vi "Vision 차선, 표지판 통합.vi"() -> ()   [LabVIEW 2016]
uses:
  <vilib>/vision/NI_Vision_Development_Module.lvlib
  <vilib>/ptbypt/NI_PtbyPt.lvlib
  <vilib>/vision/Classification.llb/IMAQ Classifier Nearest Neighbor options.ctl
panel:
  out "출력 클러스터":T1
  out "ms 타이머 값":u32
  in  "정적 횟수":u8
  in  "동적 횟수":u8
  in  "유턴 횟수":u8
  in  "Stop (F) 2":bool caption="Stop (F)"
  out "유턴이냐":bool
  in  "Type":u32(ring)=3 items=["No Selection", "Point", "Line", "Rectangle", "Oval", "Polygon", "Free", "Annulus", "Unused2", "Unused3", "Broken Line", "Free Hand Line", "Rotated Rectangle"]
  in  "ID":enum32{"External", "Internal"}(ring)
  out "동적이냐":bool
  out "정적이냐":bool
  in  "탭 컨트롤":enum32{"유턴", "동적", "정적"}(tab)
  in  "Paramaters":T3={"Preprocessing Options"={"Method"=-1, "Looking for"=1, "Threshold Range"={"Lower value"=0.0, "Upper value"=69.0}, "Threshold Limits"={"Lower value"=0.0, "Upper value"=0.0}, "Reject Border"=FALSE, "# of Erosions"=0, "Kernel Size"={"Lower value"=0, "Upper value"=0}, "Deviation Factor"=0.0}, "Nearest Neighbor Options"={"Method"=0, "Metric"=0, "k"=0}, "Particle Options"={"Scale Dependant"=FALSE, "Scale Factor"=0.0, "Symmetry Dependant"=FALSE, "Symmetry Factor"=0.0}} {"Preprocessing Options"."Deviation Factor" min=0.0; "Preprocessing Options"."Threshold Limits"."Upper value" format="%.2f"; "Preprocessing Options"."Threshold Limits"."Lower value" format="%.2f"; "Preprocessing Options"."Threshold Range"."Upper value" format="%.2f"; "Preprocessing Options"."Threshold Range"."Lower value" format="%.2f"; "Preprocessing Options"."# of Erosions" min=0; "Preprocessing Options"."Method" items=["Manual Threshold"=-1, "-"=-2, "Auto Threshold: Clustering"=0, "Auto Threshold: Entropy"=1, "Auto Threshold: Metric"=2, "Auto Threshold: Moments"=3, "Auto Threshold: Inter-class Variance"=4, "--"=-3, "Local Threshold: Niblack"=5, "Local Threshold: BG Correction"=6]; "Preprocessing Options"."Looking for" items=["Bright Objects", "Dark Objects"]; "Nearest Neighbor Options"."Method" items=["Nearest Neighbor", "K Nearest Neighbor", "Minimum Mean Distance"]; "Nearest Neighbor Options"."Metric" items=["Maximum", "Sum", "Euclidean"]; "Nearest Neighbor Options"."k" min=3}
  in  "Paramaters 2":T3={"Preprocessing Options"={"Method"=-1, "Looking for"=0, "Threshold Range"={"Lower value"=0.0, "Upper value"=45.0}, "Threshold Limits"={"Lower value"=0.0, "Upper value"=0.0}, "Reject Border"=FALSE, "# of Erosions"=0, "Kernel Size"={"Lower value"=0, "Upper value"=0}, "Deviation Factor"=0.0}, "Nearest Neighbor Options"={"Method"=0, "Metric"=0, "k"=0}, "Particle Options"={"Scale Dependant"=FALSE, "Scale Factor"=0.0, "Symmetry Dependant"=FALSE, "Symmetry Factor"=0.0}} {"Preprocessing Options"."Deviation Factor" min=0.0; "Preprocessing Options"."Threshold Limits"."Upper value" format="%.2f"; "Preprocessing Options"."Threshold Limits"."Lower value" format="%.2f"; "Preprocessing Options"."Threshold Range"."Upper value" format="%.2f"; "Preprocessing Options"."Threshold Range"."Lower value" format="%.2f"; "Preprocessing Options"."# of Erosions" min=0; "Preprocessing Options"."Method" items=["Manual Threshold"=-1, "-"=-2, "Auto Threshold: Clustering"=0, "Auto Threshold: Entropy"=1, "Auto Threshold: Metric"=2, "Auto Threshold: Moments"=3, "Auto Threshold: Inter-class Variance"=4, "--"=-3, "Local Threshold: Niblack"=5, "Local Threshold: BG Correction"=6]; "Preprocessing Options"."Looking for" items=["Bright Objects", "Dark Objects"]; "Nearest Neighbor Options"."Method" items=["Nearest Neighbor", "K Nearest Neighbor", "Minimum Mean Distance"]; "Nearest Neighbor Options"."Metric" items=["Maximum", "Sum", "Euclidean"]; "Nearest Neighbor Options"."k" min=3}
  in  "Paramaters 3":T3={"Preprocessing Options"={"Method"=-1, "Looking for"=0, "Threshold Range"={"Lower value"=0.0, "Upper value"=45.0}, "Threshold Limits"={"Lower value"=0.0, "Upper value"=0.0}, "Reject Border"=FALSE, "# of Erosions"=0, "Kernel Size"={"Lower value"=0, "Upper value"=0}, "Deviation Factor"=0.0}, "Nearest Neighbor Options"={"Method"=0, "Metric"=0, "k"=0}, "Particle Options"={"Scale Dependant"=FALSE, "Scale Factor"=0.0, "Symmetry Dependant"=FALSE, "Symmetry Factor"=0.0}} {"Preprocessing Options"."Deviation Factor" min=0.0; "Preprocessing Options"."Threshold Limits"."Upper value" format="%.2f"; "Preprocessing Options"."Threshold Limits"."Lower value" format="%.2f"; "Preprocessing Options"."Threshold Range"."Upper value" format="%.2f"; "Preprocessing Options"."Threshold Range"."Lower value" format="%.2f"; "Preprocessing Options"."# of Erosions" min=0; "Preprocessing Options"."Method" items=["Manual Threshold"=-1, "-"=-2, "Auto Threshold: Clustering"=0, "Auto Threshold: Entropy"=1, "Auto Threshold: Metric"=2, "Auto Threshold: Moments"=3, "Auto Threshold: Inter-class Variance"=4, "--"=-3, "Local Threshold: Niblack"=5, "Local Threshold: BG Correction"=6]; "Preprocessing Options"."Looking for" items=["Bright Objects", "Dark Objects"]; "Nearest Neighbor Options"."Method" items=["Nearest Neighbor", "K Nearest Neighbor", "Minimum Mean Distance"]; "Nearest Neighbor Options"."Metric" items=["Maximum", "Sum", "Euclidean"]; "Nearest Neighbor Options"."k" min=3}
  in  "탭 컨트롤 2":enum32{"유턴", "동적", "정적"}(tab)
  in  "File Path":path=path "C:/Users/SeongHyeon/Desktop/전체프로그램/Sub Vi/Sensor/Vision Reference/유턴.clf"
  in  "File Path 2":path=path "C:/Users/SeongHyeon/Desktop/전체프로그램/Sub Vi/Sensor/Vision Reference/동적.clf"
  in  "File Path 3":path=path "C:/Users/SeongHyeon/Desktop/전체프로그램/Sub Vi/Sensor/Vision Reference/정적.clf"
  in  "탭 컨트롤 3":enum32{"유턴", "동적", "정적"}(tab)
  out "유턴":T4(plugin-control)
  out "동적":T4(plugin-control)
  out "정적":T4(plugin-control)
  out "횡단보도 거리":dbl[](array[numeric])
  out "차선":dbl[][](array[numeric])
  out "Filtered image":T4(plugin-control)
  out "Original Image":T4(plugin-control)
  out "Original Image":T4(plugin-control)
  out "프레임 rate":dbl
  out "error out":errorcluster
  in  "이미지 형식":T5 items=["Grayscale (U8)", "Grayscale (I16)", "Grayscale (SGL)", "Complex (CSG)", "RGB (U32)", "HSL (U32)", "RGB (U64)", "Grayscale (U16)"]
  in  "Stop (F)":bool
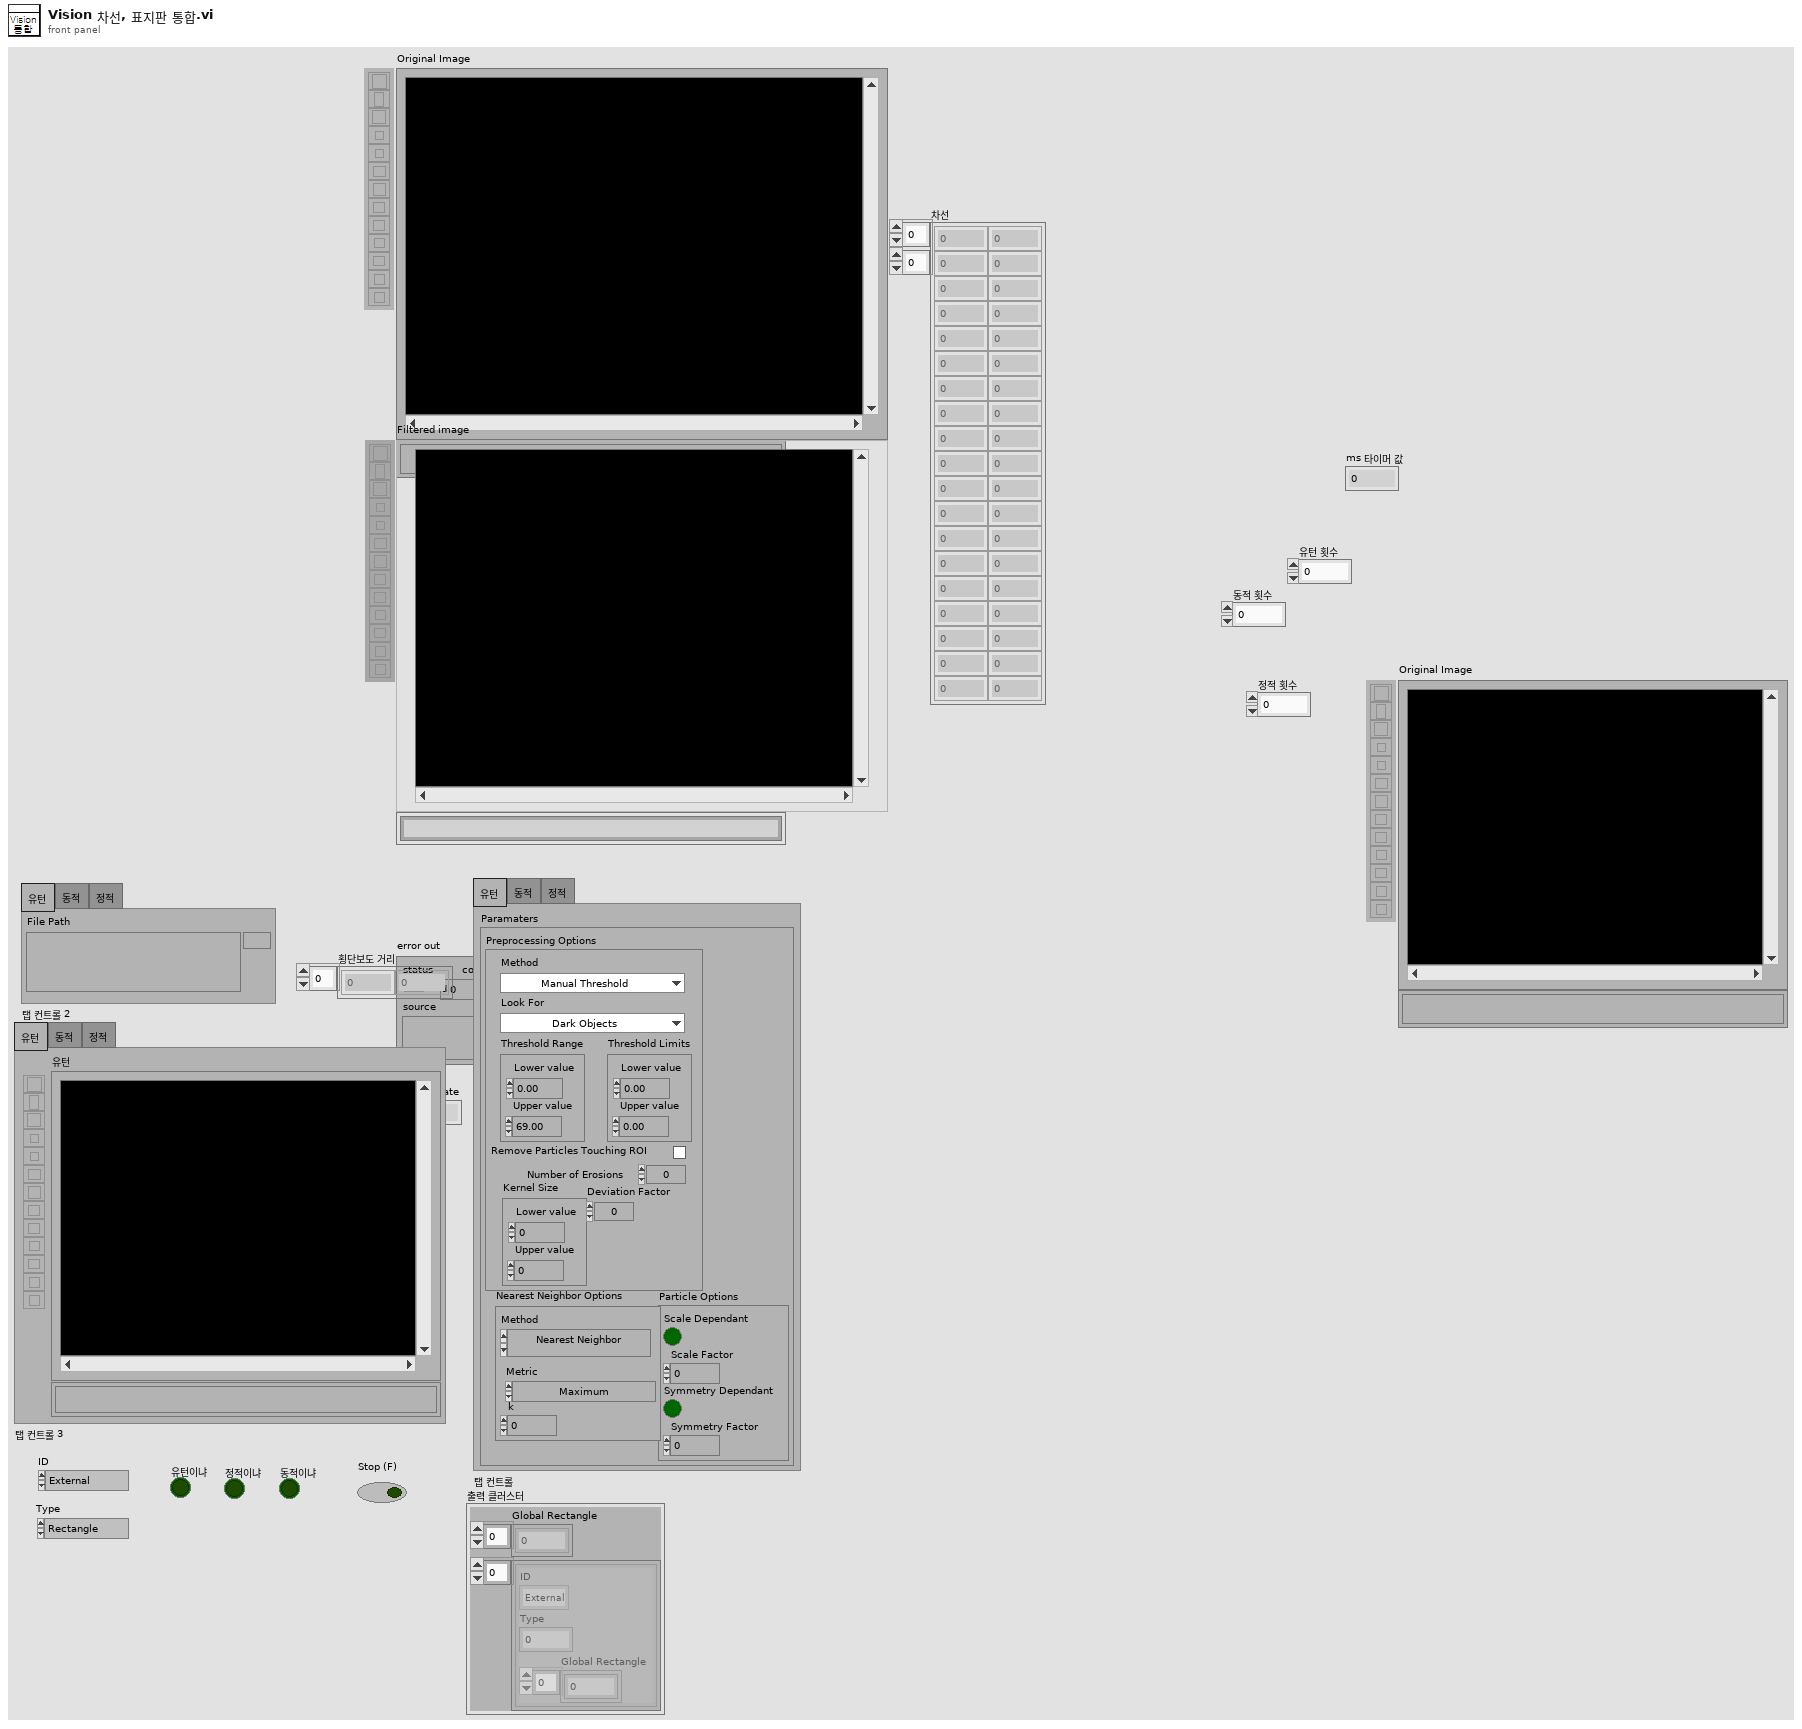
[diagram p1: front panel]
types:
  T1 = cluster{"Global Rectangle":i32[], cluster{"ID":enum32{"External", "Internal"}, "Type":u32, "Global Rectangle":i32[]}[]}
  T2 = typedef "IMAQ Classifier Nearest Neighbor options.ctl" = cluster{"Method":i32, "Metric":i32, "k":i32}
  T3 = cluster{"Preprocessing Options":cluster{"Method":i32, "Looking for":i32, "Threshold Range":cluster{"Lower value":sgl, "Upper value":sgl}, "Threshold Limits":cluster{"Lower value":sgl, "Upper value":sgl}, "Reject Border":bool, "# of Erosions":i32, "Kernel Size":cluster{"Lower value":i32, "Upper value":i32}, "Deviation Factor":dbl}, "Nearest Neighbor Options":T2, "Particle Options":cluster{"Scale Dependant":bool, "Scale Factor":sgl, "Symmetry Dependant":bool, "Symmetry Factor":sgl}}
  T4 = typedef "IMAQ Image.ctl" = refnum<image>
  T5 = typedef "Image Type" = u32
  T6 = cluster{"Position":cluster{"x":sgl, "y":sgl}, "Angle":sgl, "Scale":sgl, "Score":sgl, "Bounding Box":cluster{"x":sgl, "y":sgl}[]}[]
  T7 = cluster{"Global Rectangle":cluster{"x1Left":i32, "y1Top":i32, "x2Right":i32, "y2Bottom":i32}, "Centroid":cluster{"x":sgl, "y":sgl}, "Object Size":u32, "Score":dbl}[]
  T8 = cluster{"Position":cluster{"x":sgl, "y":sgl}, "Angle":sgl, "Scale":sgl, "Score":sgl, "Bounding Box":cluster{"x":sgl, "y":sgl}[]}
  T9 = cluster{"Global Rectangle":cluster{"x1Left":i32, "y1Top":i32, "x2Right":i32, "y2Bottom":i32}, "Centroid":cluster{"x":sgl, "y":sgl}, "Object Size":u32, "Score":dbl}
  T10 = cluster{"x1Left":i32, "y1Top":i32, "x2Right":i32, "y2Bottom":i32}
  T11 = cluster{"ID":enum32{"External", "Internal"}, "Type":u32, "Global Rectangle":i32[]}
  T12 = cluster{"ID":enum32{"External", "Internal"}, "Type":u32, "Global Rectangle":i32[]}[]
  T13 = typedef "IMAQ Classifier Session.ctl" = refnum<k1>
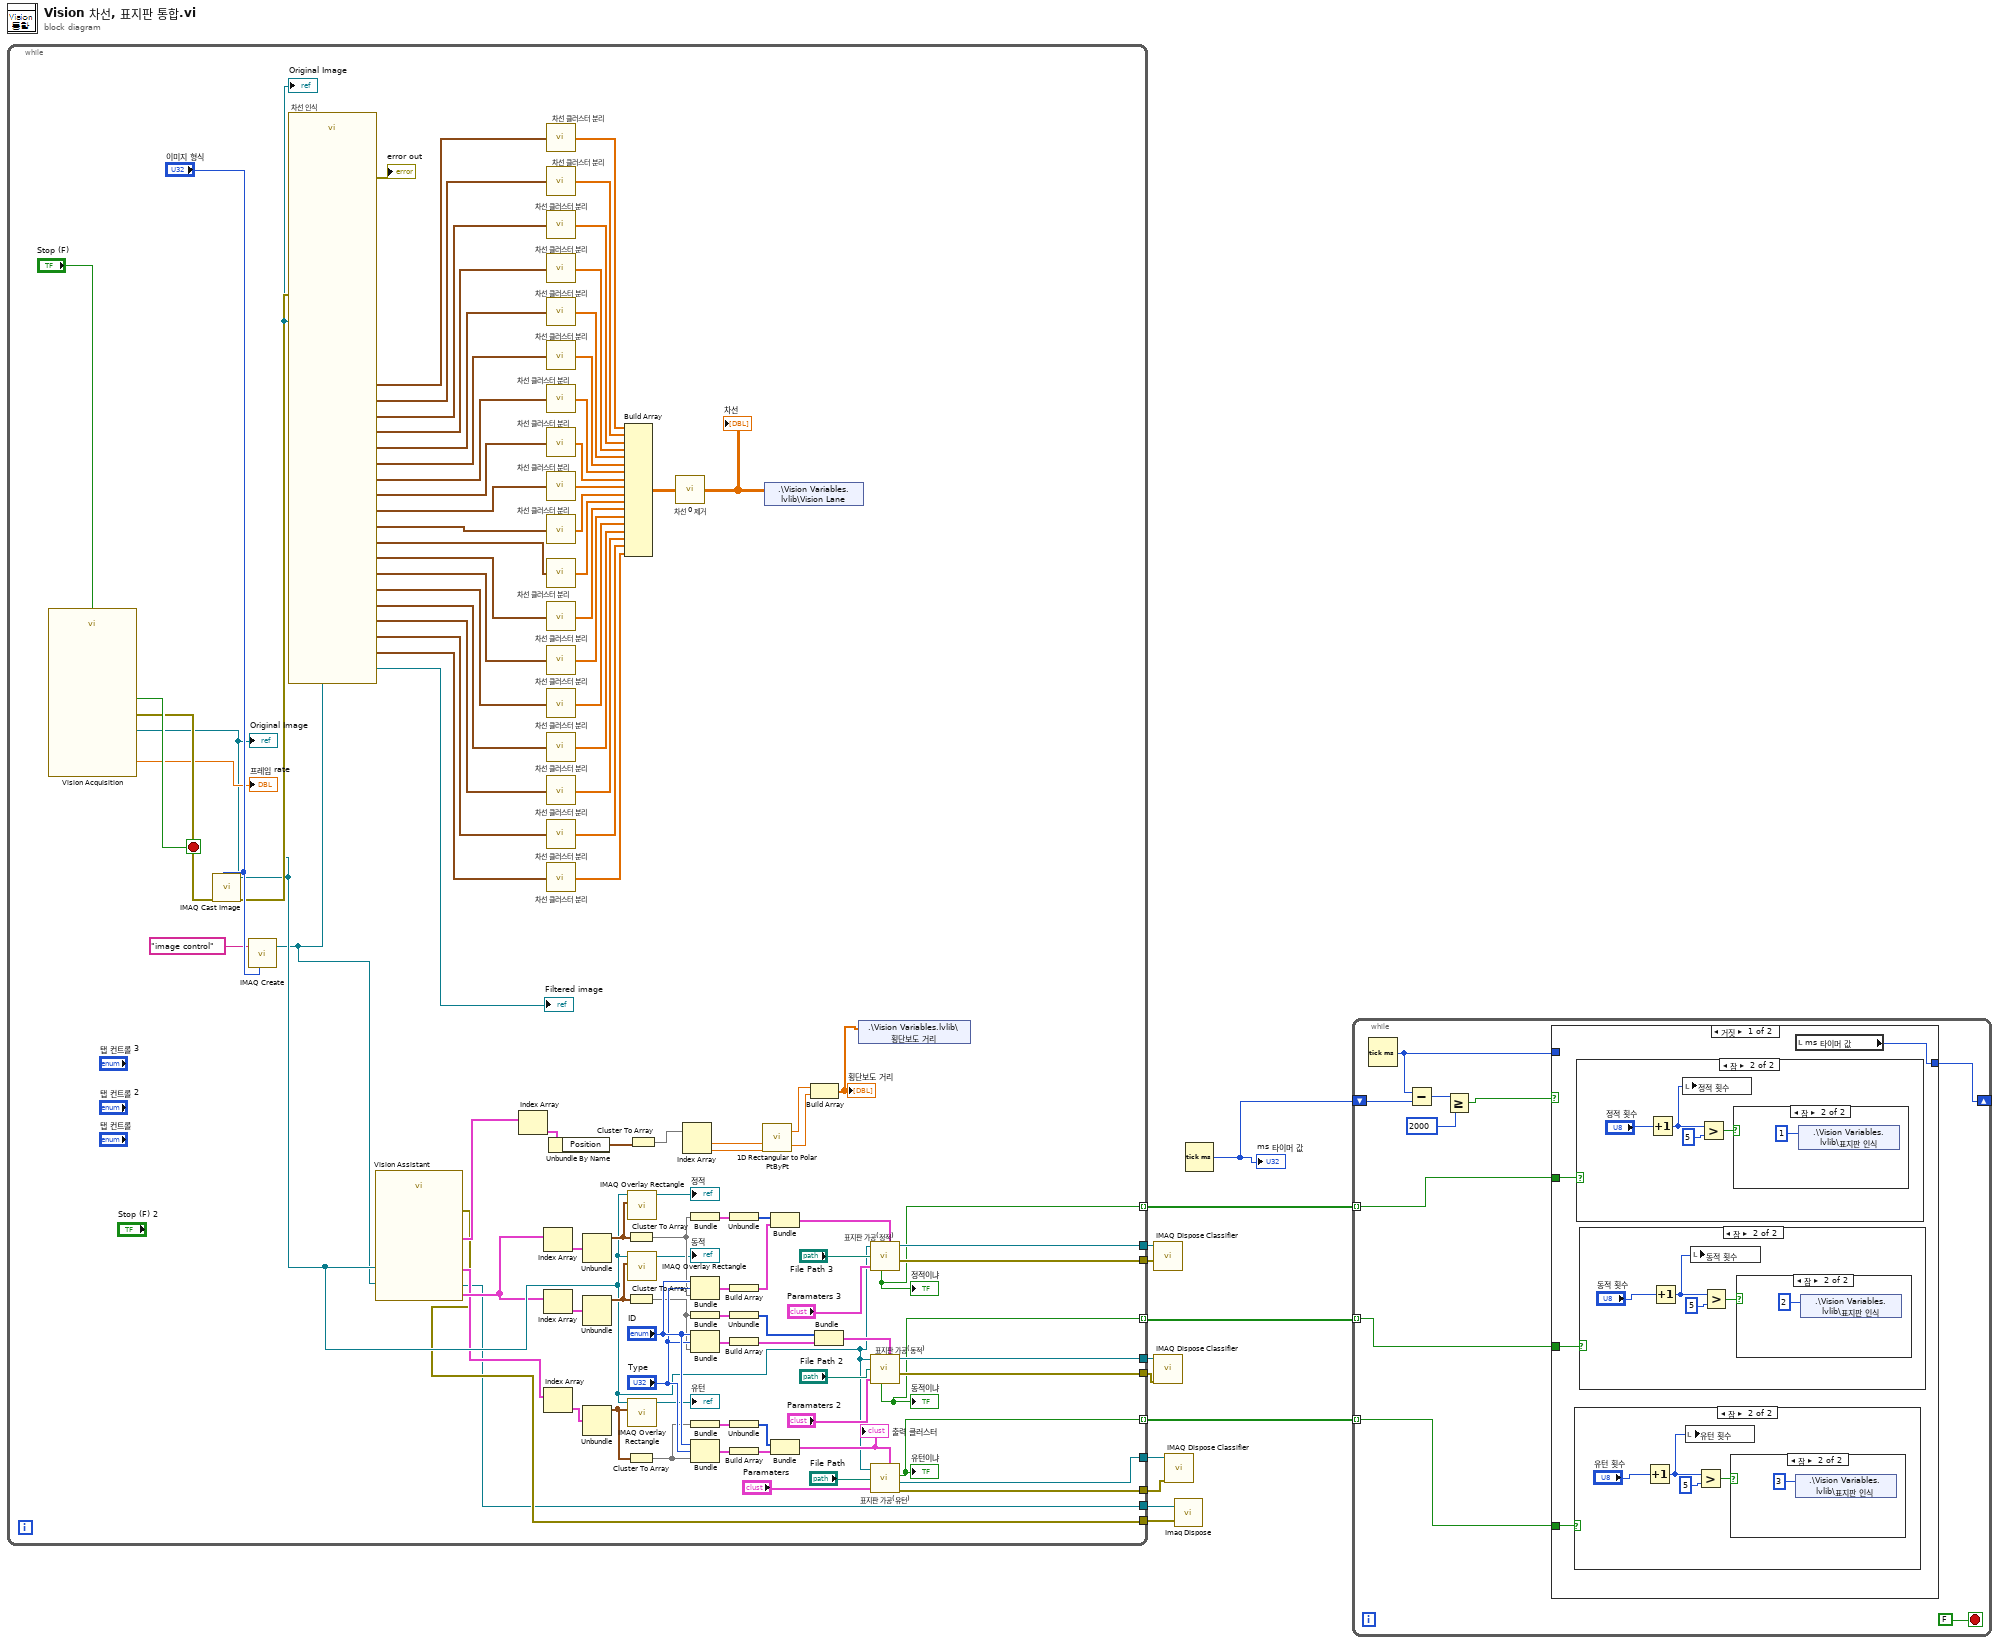
[diagram p0: block diagram]
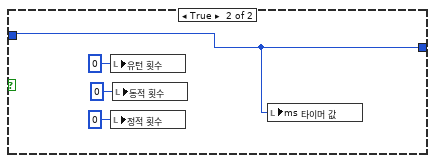
[diagram p8: hidden frame]
diagram:
  n1 = while {
    tunnel: [w24] -> w12
    tunnel: [w23] -> w11
    tunnel: [w22] -> w10
    tunnel: [w21] -> w9
    tunnel: [w20] -> w8
    tunnel: [w19] -> w7
    tunnel: [w18] -> w2
    tunnel: [w16] -> w5 mode=indexing
    tunnel: [w15] -> w4 mode=indexing
    tunnel: [w14] -> w3 mode=indexing
    tunnel: [w13] -> w1
    stop <- w118 stop-if-true
    n2 = call "Vision Acquisition"("Stop (F)"="Stop (F)") -> ("Image Out"=w73:T4, "Frame Rate"=→"프레임 rate":dbl, "Stopped"=w118:bool, "error out"=w115:errorcluster)  [unwired: 23 in]
    "Original Image" <- w73
    n3 = call "IMAQ Cast Image"("Image Type"="이미지 형식", "error in (no error)"=w115, "Image Src"=w73) -> ("error out"=w114:errorcluster, "Image Dst Out"=w29:T4)  [unwired: 7 in]
    "Original Image" <- w29
    n4 = call "IMAQ Create"("Image Name"="image control", "Image Type"="이미지 형식") -> ("New Image"=w28:T4)  [unwired: 3 in, 1 out]
    n5 = call "차선 인식"("Image In"=w29, "Image Dst"=w28, "error in"=w114) -> ("Edges Coordinates (calibrated) (Edge Detector 21)"=w92:cluster{"X":sgl, "Y":sgl}[], "Edges Coordinates (calibrated) (Edge Detector 20)"=w93:cluster{"X":sgl, "Y":sgl}[], "Edges Coordinates (calibrated) (Edge Detector 19)"=w94:cluster{"X":sgl, "Y":sgl}[], "Edges Coordinates (calibrated) (Edge Detector 18)"=w95:cluster{"X":sgl, "Y":sgl}[], "Edges Coordinates (calibrated) (Edge Detector 17)"=w96:cluster{"X":sgl, "Y":sgl}[], "Edges Coordinates (calibrated) (Edge Detector 16)"=w97:cluster{"X":sgl, "Y":sgl}[], "Edges Coordinates (calibrated) (Edge Detector 15)"=w98:cluster{"X":sgl, "Y":sgl}[], "Edges Coordinates (calibrated) (Edge Detector 13)"=w99:cluster{"X":sgl, "Y":sgl}[], "Edges Coordinates (calibrated) (Edge Detector 12)"=w100:cluster{"X":sgl, "Y":sgl}[], "Edges Coordinates (calibrated) (Edge Detector 11)"=w101:cluster{"X":sgl, "Y":sgl}[], "Edges Coordinates (calibrated) (Edge Detector 10)"=w102:cluster{"X":sgl, "Y":sgl}[], "Edges Coordinates (calibrated) (Edge Detector 8)"=w103:cluster{"X":sgl, "Y":sgl}[], "Edges Coordinates (calibrated) (Edge Detector 7)"=w104:cluster{"X":sgl, "Y":sgl}[], "Edges Coordinates (calibrated) (Edge Detector 5)"=w105:cluster{"X":sgl, "Y":sgl}[], "Image Out"=→"Filtered image":T4, "Edges Coordinates (calibrated) (Edge Detector 1)"=w111:cluster{"X":sgl, "Y":sgl}[], "Edges Coordinates (calibrated) (Edge Detector 2)"=w109:cluster{"X":sgl, "Y":sgl}[], "Edges Coordinates (calibrated) (Edge Detector 3)"=w107:cluster{"X":sgl, "Y":sgl}[], "Edges Coordinates (calibrated) (Edge Detector 4)"=w106:cluster{"X":sgl, "Y":sgl}[], "error out"=→"error out":errorcluster)  [unwired: 3 in, 2 out]
    n6 = call "Vision Assistant"("Image In"=w29, "Image Dst"=w28) -> ("Image Out"=w13:T4, "Calibrated Matches (Pattern Matching 1)"=w27:T6, "Shape Report (Shape Matching 1)"=w26:T7, "Shape Report (Shape Matching 2)"=w25:T7, "error out"=w18:errorcluster)  [unwired: 21 in]
    n7 = Index Array(array=w27) -> (element=w65:T8)  [unwired: 1 in]
    n8 = Index Array(array=w26) -> (element=w54:T9)  [unwired: 1 in]
    n9 = Index Array(array=w26) -> (element=w41:T9)  [unwired: 1 in]
    n10 = Index Array(array=w25) -> (element=w30:T9)  [unwired: 1 in]
    n11 = call "차선 클러스터 분리.vi"("배열"=w111) -> ("R, Theta"=w110:dbl[])
    n12 = call "차선 클러스터 분리.vi"("배열"=w109) -> ("R, Theta"=w108:dbl[])
    n13 = call "차선 클러스터 분리.vi"("배열"=w107) -> ("R, Theta"=w91:dbl[])
    n14 = call "차선 클러스터 분리.vi"("배열"=w106) -> ("R, Theta"=w90:dbl[])
    n15 = call "차선 클러스터 분리.vi"("배열"=w105) -> ("R, Theta"=w89:dbl[])
    n16 = call "차선 클러스터 분리.vi"("배열"=w104) -> ("R, Theta"=w88:dbl[])
    n17 = call "차선 클러스터 분리.vi"("배열"=w103) -> ("R, Theta"=w87:dbl[])
    n18 = call "차선 클러스터 분리.vi"("배열"=w102) -> ("R, Theta"=w86:dbl[])
    n19 = call "차선 클러스터 분리.vi"("배열"=w101) -> ("R, Theta"=w85:dbl[])
    n20 = call "차선 클러스터 분리.vi"("배열"=w100) -> ("R, Theta"=w84:dbl[])
    n21 = call "차선 클러스터 분리.vi"("배열"=w99) -> ("R, Theta"=w83:dbl[])
    n22 = call "차선 클러스터 분리.vi"("배열"=w98) -> ("R, Theta"=w82:dbl[])
    n23 = call "차선 클러스터 분리.vi"("배열"=w97) -> ("R, Theta"=w81:dbl[])
    n24 = call "차선 클러스터 분리.vi"("배열"=w96) -> ("R, Theta"=w80:dbl[])
    n25 = call "차선 클러스터 분리.vi"("배열"=w95) -> ("R, Theta"=w78:dbl[])
    n26 = call "차선 클러스터 분리.vi"("배열"=w94) -> ("R, Theta"=w77:dbl[])
    n27 = call "차선 클러스터 분리.vi"("배열"=w93) -> ("R, Theta"=w76:dbl[])
    n28 = call "차선 클러스터 분리.vi"("배열"=w92) -> ("R, Theta"=w75:dbl[])
    n29 = Unbundle By Name(w65) -> ("Position"=w66:cluster{"x":sgl, "y":sgl})
    n30 = Unbundle(w54) -> ("Global Rectangle"=w61:T10)  [unwired: 3 out]
    n31 = Unbundle(w41) -> ("Global Rectangle"=w48:T10)  [unwired: 3 out]
    n32 = Unbundle(w30) -> ("Global Rectangle"=w37:T10)  [unwired: 3 out]
    n33 = Build Array(w110, w108, w91, w90, w89, w88, w87, w86, w85, w84, w83, w82, w81, w80, w78, w77, w76, w75) -> (w74:dbl[][])
    n34 = Cluster To Array(cluster=w61) -> (array=w55:i32[])
    n35 = Cluster To Array(cluster=w48) -> (array=w42:i32[])
    n36 = Cluster To Array(cluster=w37) -> (array=w31:i32[])
    n37 = call "IMAQ Overlay Rectangle"("Rectangle"=w61, "Image"=w29) -> ("Image Out"=→"정적":T4)  [unwired: 8 in, 1 out]
    n38 = call "IMAQ Overlay Rectangle"("Rectangle"=w48, "Image"=w29) -> ("Image Out"=→"동적":T4)  [unwired: 8 in, 1 out]
    n39 = call "IMAQ Overlay Rectangle"("Rectangle"=w37, "Image"=w29) -> ("Image Out"=→"유턴":T4)  [unwired: 8 in, 1 out]
    n40 = Cluster To Array(cluster=w66) -> (array=w67:sgl[])
    n41 = call "차선 0 제거.vi"("추가된 배열"=w74) -> ("추가된 배열 2"=w72:dbl[][])
    "차선" <- w72
    n42 = Index Array(array=w67) -> (element #1=w68:sgl, element #2=w69:sgl)  [unwired: 2 in]
    n43 = Bundle("Global Rectangle"=w55) -> (w56:cluster{"Global Rectangle":i32[]})  [unwired: 1 in]
    n44 = Bundle("ID"="ID", "Type"="Type", "Global Rectangle"=w55) -> (w58:T11)  [unwired: 1 in]
    n45 = Bundle("Global Rectangle"=w42) -> (w43:cluster{"Global Rectangle":i32[]})  [unwired: 1 in]
    n46 = Bundle("ID"="ID", "Type"="Type", "Global Rectangle"=w42) -> (w45:T11)  [unwired: 1 in]
    n47 = Bundle("Global Rectangle"=w31) -> (w32:cluster{"Global Rectangle":i32[]})  [unwired: 1 in]
    n48 = Bundle("ID"="ID", "Type"="Type", "Global Rectangle"=w31) -> (w34:T11)  [unwired: 1 in]
    n49 = Unbundle(w56) -> ("Global Rectangle"=w57:i32[])
    n50 = Build Array(w58) -> (w59:T12)
    n51 = Unbundle(w43) -> ("Global Rectangle"=w44:i32[])
    n52 = Build Array(w45) -> (w46:T12)
    n53 = Unbundle(w32) -> ("Global Rectangle"=w33:i32[])
    n54 = Build Array(w34) -> (w35:T12)
    n55 = call <vilib>:"1D Rectangular to Polar PtByPt.vi"("y"=w69, "x"=w68) -> ("phase"=w71:dbl, "magnitude"=w70:dbl)
    n56 = shared-variable ".\\Vision Variables.lvlib\\Vision Lane"(w72) -> ()  [unwired: 1 in, 1 out]
    n57 = Bundle("Global Rectangle"=w57, w59) -> (w62:T1)  [unwired: 1 in]
    n58 = Bundle("Global Rectangle"=w33, w35) -> (w40:T1)  [unwired: 1 in]
    "출력 클러스터" <- w40
    n59 = Build Array(w70, w71) -> (w17:dbl[])
    "횡단보도 거리" <- w17
    n60 = Bundle("Global Rectangle"=w44, w46) -> (w51:T1)  [unwired: 1 in]
    n61 = shared-variable ".\\Vision Variables.lvlib\\횡단보도 거리"(w17) -> ()  [unwired: 1 in, 1 out]
    n62 = call "표지판 가공(정적).vi"("Image 2"=w29, "File Path"="File Path 3", "Paramaters"="Paramaters 3", "ROI Descriptor (Particle Classification 1)"=w62) -> ("주차냐"=w16:bool, "Classifier Session (dup)"=w24:T13, "error out"=w23:errorcluster)  [unwired: 3 in, 1 out]
    "정적이냐" <- w16
    n63 = call "표지판 가공(동적).vi"("Image 2"=w29, "File Path"="File Path 2", "Paramaters"="Paramaters 2", "ROI Descriptor (Particle Classification 1)"=w51) -> ("주차냐"=w15:bool, "Classifier Session (dup)"=w22:T13, "error out"=w21:errorcluster)  [unwired: 3 in, 1 out]
    "동적이냐" <- w15
    n64 = call "표지판 가공(유턴).vi"("Image 2"=w29, "File Path"="File Path", "Paramaters"="Paramaters", "ROI Descriptor (Particle Classification 1)"=w40) -> ("주차냐"=w14:bool, "Classifier Session (dup)"=w20:T13, "error out"=w19:errorcluster)  [unwired: 3 in, 1 out]
    "유턴이냐" <- w14
  }
  n65 = call "IMAQ Dispose Classifier"("error in (no error)"=w11, "Classifier Session"=w12) -> ()  [unwired: 9 in, 1 out]
  n66 = call "IMAQ Dispose Classifier"("error in (no error)"=w9, "Classifier Session"=w10) -> ()  [unwired: 9 in, 1 out]
  n67 = call "IMAQ Dispose Classifier"("error in (no error)"=w7, "Classifier Session"=w8) -> ()  [unwired: 9 in, 1 out]
  n68 = call "Imaq Dispose"("Image"=w1, "error in (no error)"=w2) -> ()  [unwired: 4 in, 1 out]
  n69 = Tick Count (ms)() -> (millisecond timer value=w6:u32)
  "ms 타이머 값" <- w6
  n70 = while {
    shift-right: [w123] -> _
    shift-left: w6 -> [w129]
    tunnel: w5 -> [w122] mode=indexing
    tunnel: w3 -> [w120] mode=indexing
    tunnel: w4 -> [w121] mode=indexing
    stop <- FALSE stop-if-true
    n71 = Tick Count (ms)() -> (millisecond timer value=w124:u32)
    n72 = Subtract(x=w124, y=w129) -> (x-y=w128:u32)
    n73 = Greater Or Equal?(x=w128, y=u32 2000) -> (x >= y?=w125:bool)
    n74 = case shown="거짓" w125 {
      tunnel: w122 -> [w133 _]
      tunnel: w121 -> [w132 _]
      tunnel: w120 -> [w131 _]
      tunnel: w124 -> [_ w149]
      tunnel: [w130 w149] -> w123
      frame False {
        n75 = case shown="참" w131 {
          frame False {
          }
          frame True {
            n76 = Increment(x="유턴 횟수") -> (x+1=w135:u8)
            n77 = local write "유턴 횟수"(w135) -> ()
            n78 = Greater?(x=w135, y=u8 5) -> (0:w136:bool)
            n79 = case shown="참" w136 {
              frame False {
              }
              frame True {
                n80 = shared-variable ".\\Vision Variables.lvlib\\표지판 인식"(u8 3 ("표지판 인식")) -> ()  [unwired: 1 in, 1 out]
              }
            }
          }
        }
        n81 = case shown="참" w133 {
          frame False {
          }
          frame True {
            n82 = Increment(x="정적 횟수") -> (x+1=w146:u8)
            n83 = local write "정적 횟수"(w146) -> ()
            n84 = Greater?(x=w146, y=u8 5) -> (0:w145:bool)
            n85 = case shown="참" w145 {
              frame False {
              }
              frame True {
                n86 = shared-variable ".\\Vision Variables.lvlib\\표지판 인식"(u8 1 ("표지판 인식")) -> ()  [unwired: 1 in, 1 out]
              }
            }
          }
        }
        n87 = case shown="참" w132 {
          frame False {
          }
          frame True {
            n88 = Increment(x="동적 횟수") -> (x+1=w139:u8)
            n89 = local write "동적 횟수"(w139) -> ()
            n90 = Greater?(x=w139, y=u8 5) -> (0:w141:bool)
            n91 = case shown="참" w141 {
              frame False {
              }
              frame True {
                n92 = shared-variable ".\\Vision Variables.lvlib\\표지판 인식"(u8 2 ("표지판 인식")) -> ()  [unwired: 1 in, 1 out]
              }
            }
          }
        }
        n93 = local read "ms 타이머 값"() -> (w130:u32)
      }
      frame True {
        n94 = local write "유턴 횟수"(u8 0 ("유턴 횟수")) -> ()
        n95 = local write "정적 횟수"(u8 0 ("유턴 횟수")) -> ()
        n96 = local write "동적 횟수"(u8 0 ("유턴 횟수")) -> ()
        n97 = local write "ms 타이머 값"(w149) -> ()
      }
    }
  }
